vi "Autonomous Independent.vi"() -> ()   [LabVIEW 2019]
doc: "This VI is called when autonomous begins, and will automatically be terminated when autonomous ends. You can carry out timed or sensor driven robot movement independently without needing to return to the caller."
uses:
  <vilib>/Rock Robotics/WPI/Utilities/WPI_GetSetVariantRefNum.vi
  <vilib>/Rock Robotics/Network Tables/NT Write Numeric Array.vi
  <vilib>/Rock Robotics/WPI/RobotDrive/WPI_RobotDriveArcadeDrive_Standard(NoSaturation).vi
  <vilib>/Rock Robotics/Network Tables/NT Read String.vi
  <vilib>/Rock Robotics/WPI/Ultrasonic/WPI_SonarSRF04DigitalRefNum Registry Get.vi
  <vilib>/Rock Robotics/WPI/Ultrasonic/WPI_SonarSRF04DigitalGetRange.vi
  <vilib>/Rock Robotics/WPI/Ultrasonic/WPI_UltrasonicRangeUnits.ctl
panel:
  out "Ultrasonic 2":dbl
  out "Ultrasonic":dbl
  out "Degrees 2":dbl(knob) scale=0.0..360.0
  out "Degrees":dbl(knob) scale=0.0..360.0
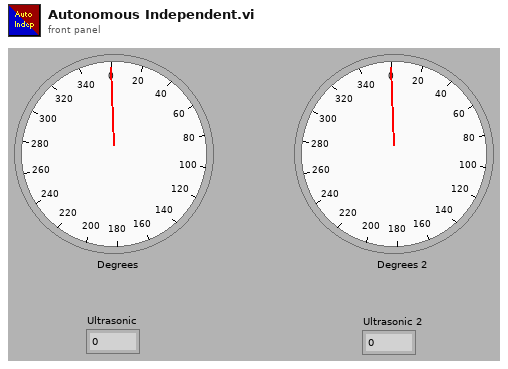
[diagram p1: front panel]
types:
  T1 = typedef "WPI_JoystickDevRef.ctl" = cluster{"Device":T2}
  T2 = typedef "WPI_JoystickDeviceEnum.ctl" = enum16{"USB 0", "USB 1", "USB 2", "USB 3", "USB 4", "USB 5"}
  T3 = typedef "WPI_UltrasonicRangeUnits.ctl" = enum16{"inches", "mm"}
  T4 = typedef "WPI_RobotDriveDevRef.ctl" = cluster{"DevStatus":errorcluster, "Motors[]":T5[], "Square Inputs":bool, "Max Output":dbl}
  T5 = typedef "WPI_MotorControlDeviceRef.ctl" = cluster{"DeviceStatus":errorcluster, "Type":T6, "PWM":cluster{"PWM Channel":T7, "DeadBand":T8}, "CAN":cluster{"Device Number":u8, "SetOutput VI Ref":variant, "GetOutput VI Ref":variant, "Enable VI Ref":variant, "Disable VI Ref":variant, "Data":variant}, "Invert":bool, "DIO PWM":cluster{"PWM \"Enable\" Channel":T7, "DIOChannel":T9, "PWM Rate":dbl}}
  T6 = typedef "WPI_MotorControlType.ctl" = enum16{"PWM", "CAN", "DIO PWM"}
  T7 = typedef "FPGA_DIOPWMChannel.ctl" = enum8{"PWM 0", "PWM 1", "PWM 2", "PWM 3", "PWM 4", "PWM 5", "PWM 6", "PWM 7", "PWM 8", "PWM 9", "PWM MXP 0", "PWM MXP 1", "PWM MXP 2", "PWM MXP 3", "PWM MXP 4", "PWM MXP 5", "PWM MXP 6", "PWM MXP 7", "PWM MXP 8", "PWM MXP 9", "Invalid"}
  T8 = typedef "WPI_PWMDeadband.ctl" = cluster{"Name":string, "maxPositivePwm":i32, "minPositivePwm":i32, "centerPwm":i32, "maxNegativePwm":i32, "minNegativePwm":i32, "angularRange":u16}
  T9 = typedef "FPGA_DIOChannel.ctl" = enum8{"DIO 0", "DIO 1", "DIO 2", "DIO 3", "DIO 4", "DIO 5", "DIO 6", "DIO 7", "DIO 8", "DIO 9", "DIO MXP 0", "DIO MXP 1", "DIO MXP 2", "DIO MXP 3", "DIO MXP 4", "DIO MXP 5", "DIO MXP 6", "DIO MXP 7", "DIO MXP 8", "DIO MXP 9", "DIO MXP 10", "DIO MXP 11", "DIO MXP 12", "DIO MXP 13", "DIO MXP 14", "DIO MXP 15", "SPI Port CS1", "SPI Port CS2", "SPI Port CS3", "SPI Port MISO", "SPI Port MOSI", "Invalid"}
  T10 = typedef "WPI_I2CDevRef.ctl" = cluster{"DevStatus":errorcluster, "Device Address":u8, "Handle":i32, "I2C Bus":T11}
  T11 = typedef "i2c_bus.ctl" = enum16{"I2C On-Board", "I2C MXP", "Invalid"}
  T12 = typedef "WPI_UltrasonicDeviceRef.ctl" = cluster{"DevStatus":errorcluster, "Ping Channel":T9, "Echo Channel":T9, "CntIndex":T13}
  T13 = typedef "FPGA_CounterCtrSystemIndex.ctl" = enum8{"Ctr 0", "Ctr 1", "Ctr 2", "Ctr 3", "Ctr 4", "Ctr 5", "Ctr 6", "Ctr 7", "Invalid"}
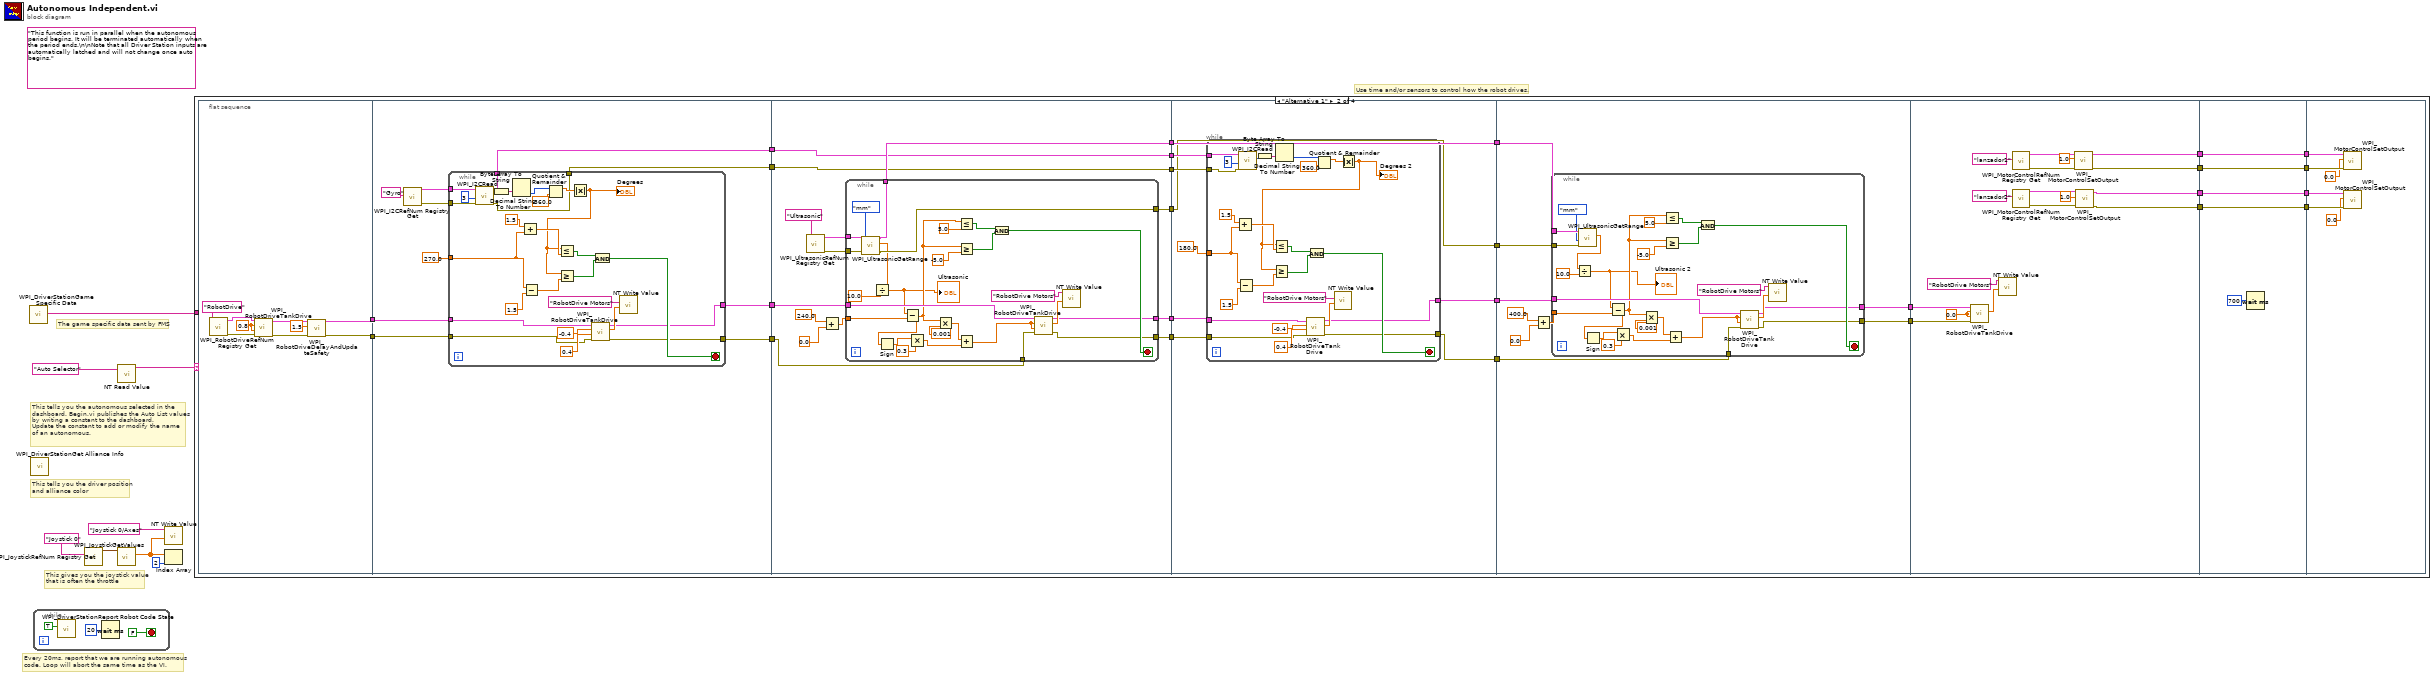
[diagram p0: block diagram]
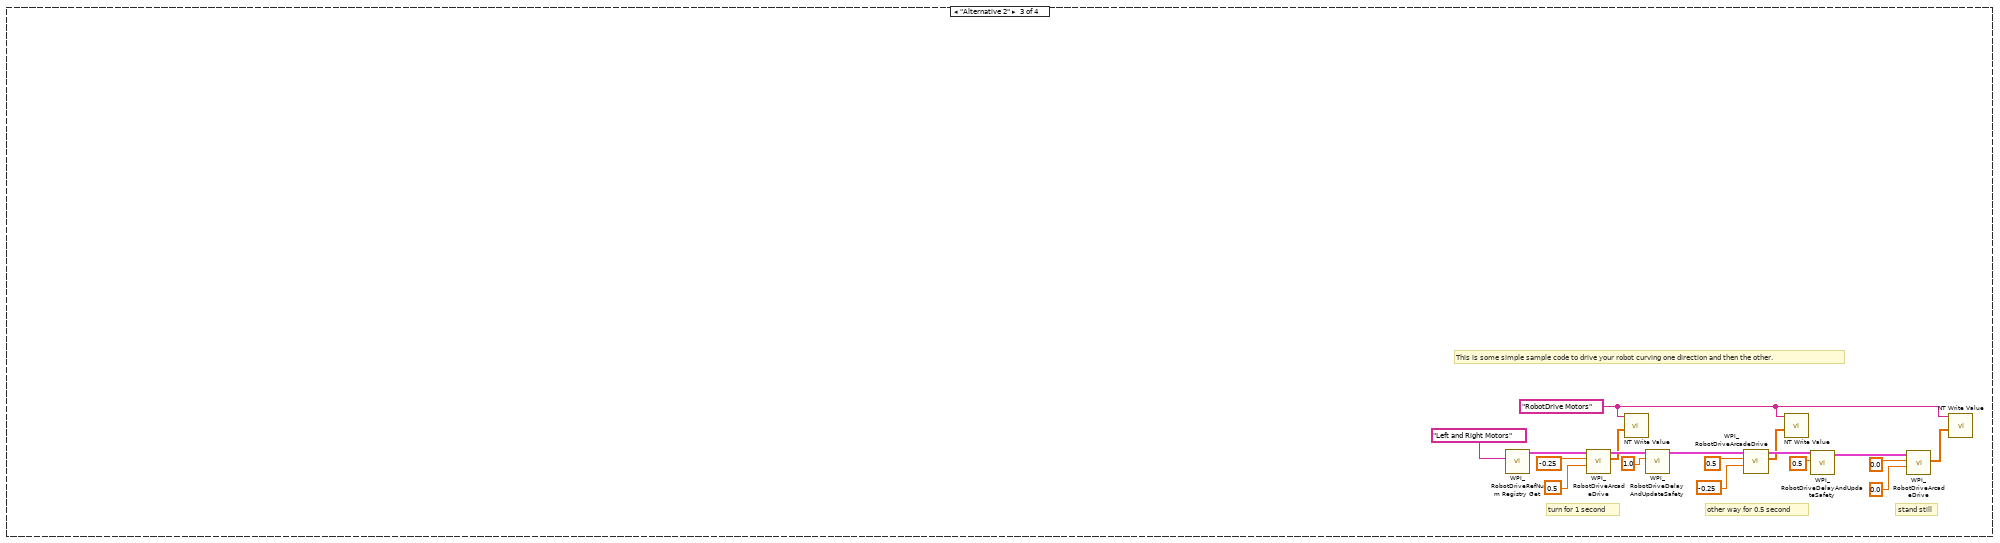
[diagram p3: hidden frame]
diagram:
  (unwired) "This function is run in parallel when the autonomous period begins. It will be terminated automatically when the period ends.\n\nNote that all Driver Station inputs are automatically latched and will not change once auto begins."
  # "The game specific data sent by FMS"
  # "This tells you the autonomous selected in the \ndashboard. Begin.vi publishes the Auto List values\nby writing a constant to the dashboard.\nUpdate the constant to add or modify the name\nof an autonomous."
  # "Every 20ms, report that we are running autonomous\ncode. Loop will abort the same time as the VI."
  # "This gives you the joystick value\nthat is often the throttle"
  # "Use time and/or sensors to control how the robot drives."
  # "This tells you the driver position\nand alliance color"
  n1 = call <vilib>:"WPI_DriverStationGame Specific Data.vi"() -> ("Game Specific Data"=w1:string)  [unwired: 11 in]
  n2 = call <vilib>:"WPI_DriverStationGet Alliance Info.vi"() -> ()  [unwired: 12 out]
  n3 = while {
    stop <- FALSE stop-if-true
    n4 = call <vilib>:"WPI_DriverStationReport Robot Code State.vi"("Autonomous"=TRUE) -> ()  [unwired: 10 in, 1 out]
    n5 = Wait (ms)(milliseconds to wait=u32 20) -> ()  [unwired: 1 out]
  }
  n6 = call <vilib>:"WPI_JoystickRefNum Registry Get.vi"("refnum name"="Joystick 0") -> ("JoystickDevRef"=w7:T1)  [unwired: 1 in, 9 out]
  n7 = call <vilib>:"WPI_JoystickGetValues.vi"("JoystickDevRef"=w7) -> ("Axes"=w3:dbl[])  [unwired: 6 in, 4 out]
  n8 = call-poly <vilib>:"NT Read Value.vi"("Name"="Auto Selector") -> ("String"=w4:string)  [unwired: 9 in, 1 out]
  n9 = call-poly <vilib>:"NT Write Value.vi"("Numeric Array"=w3, "Name"="Joystick 0/Axes") -> ()  [unwired: 9 in, 1 out]
  n10 = Index Array(array=w3, index=2) -> ()  [unwired: 1 out]
  n11 = case shown="\"Alternative 1\"" w4 {
    tunnel: w1 -> [_ _ _ _]
    frame Default {
      # "You can put your main auto here, or you can right-click on the case and make any\nother frame be the default case."
      # "This is the frame that will execute if no selection is made, or if it is not recognized"
    }
    frame "Alternative 1" {
      n12 = flat-sequence {
        tunnel: [w38] -> w15
        tunnel: [w39] -> w14
        tunnel: [w55] -> w37
        tunnel: [w54] -> w36
        tunnel: w15 -> [w50]
        tunnel: w14 -> [w49]
        tunnel: [w48] -> w13
        tunnel: [w47] -> w12
        tunnel: w37 -> [w91]
        tunnel: w36 -> [w90]
        tunnel: [w89] -> w35
        tunnel: [w88] -> w34
        tunnel: [w85] -> w33
        tunnel: [w84] -> w32
        tunnel: [w87] -> w31
        tunnel: [w86] -> w30
        tunnel: w13 -> [w85]
        tunnel: w12 -> [w84]
        tunnel: w35 -> [w133]
        tunnel: w34 -> [w132]
        tunnel: w33 -> [w130]
        tunnel: w32 -> [w129]
        tunnel: [w128] -> w29
        tunnel: [w127] -> w28
        tunnel: [w126] -> w27
        tunnel: w31 -> [w126]
        tunnel: [w125] -> w26
        tunnel: w30 -> [w125]
        tunnel: w29 -> [w167]
        tunnel: w28 -> [w163]
        tunnel: w27 -> [w162]
        tunnel: w26 -> [w161]
        tunnel: [w160] -> w25
        tunnel: [w159] -> w24
        tunnel: w25 -> [w199]
        tunnel: w24 -> [w198]
        tunnel: [w196] -> w23
        tunnel: [w195] -> w22
        tunnel: [w194] -> w21
        tunnel: [w193] -> w20
        tunnel: [w213] -> w19
        tunnel: w23 -> [w213]
        tunnel: [w212] -> w18
        tunnel: w22 -> [w212]
        tunnel: [w211] -> w17
        tunnel: w21 -> [w211]
        tunnel: [w210] -> w16
        tunnel: w20 -> [w210]
        tunnel: w19 -> [w220]
        tunnel: w18 -> [w219]
        tunnel: w17 -> [w218]
        tunnel: w16 -> [w217]
        frame #0 {
          w43 = 0.8 ("Left axis value")
          n13 = call <vilib>:"WPI_RobotDriveRefNum Registry Get.vi"("refnum name"="RobotDrive") -> ("error out"=w41:errorcluster, "RobotDriveDevRef"=w42:T4)  [unwired: 9 in]
          n14 = call <vilib>:"WPI_RobotDriveTankDrive.vi"("error in (no error)"=w41, "Right axis value"=w43, "Left axis value"=w43, "RobotDriveDevRef"=w42) -> ("error out"=w44:errorcluster, "RobotDriveDevRef"=w45:T4)  [unwired: 5 in, 1 out]
          n15 = call <vilib>:"WPI_RobotDriveDelayAndUpdateSafety.vi"("error in (no error)"=w44, "Delay (s)"=1.5, "RobotDriveDevRef"=w45) -> ("error out"=w38:errorcluster, "RobotDriveDevRef 2"=w39:T4)  [unwired: 7 in]
        }
        frame #1 {
          n16 = call <vilib>:"WPI_I2CRefNum Registry Get.vi"("refnum name"="Gyro") -> ("error out"=w52:errorcluster, "I2CDevRef"=w51:T10)  [unwired: 9 in]
          n17 = while {
            tunnel: 270.0 ("y") -> [w76]
            tunnel: [w69] -> w55
            tunnel: [w68] -> w54
            tunnel: w52 -> [w65]
            tunnel: w51 -> [w64]
            tunnel: w50 -> [w60]
            tunnel: w49 -> [w59]
            tunnel: [w58] -> w48
            tunnel: [w57] -> w47
            stop <- w79 stop-if-true
            n18 = call <vilib>:"WPI_I2CRead.vi"("error in (no error)"=w65, "I2CBytesToRead"=u8 3, "I2CDevRef"=w64) -> ("error out"=w57:errorcluster, "Data Out"=w62:u8[], "I2CDevRef"=w58:T10)  [unwired: 6 in]
            n19 = Byte Array To String(unsigned byte array=w62) -> (string=w66:string)
            n20 = Decimal String To Number(string=w66) -> (number=w61:i32)  [unwired: 2 in, 1 out]
            n21 = Add(x=1.5 ("y"), y=w76) -> (x+y=w72:dbl)
            n22 = Subtract(x=w76, y=1.5 ("x")) -> (x-y=w73:dbl)
            n23 = Quotient & Remainder(x=w61, y=360.0) -> (x-y*floor(x/y)=w70:dbl)  [unwired: 1 out]
            n24 = Absolute Value(x=w70) -> (abs(x)=w67:dbl)
            "Degrees" <- w67
            n25 = Less Or Equal?(x=w67, y=w72) -> (x <= y?=w74:bool)
            n26 = Greater Or Equal?(x=w67, y=w73) -> (x >= y?=w75:bool)
            n27 = call <vilib>:"WPI_RobotDriveTankDrive.vi"("error in (no error)"=w60, "Right axis value"=0.4 ("X axis value"), "Left axis value"=-0.4 ("X axis value"), "RobotDriveDevRef"=w59) -> ("error out"=w68:errorcluster, "Motor Values"=w83:dbl[], "RobotDriveDevRef"=w69:T4)  [unwired: 5 in]
            n28 = And(x=w74, y=w75) -> (x .and. y?=w79:bool)
            n29 = call-poly <vilib>:"NT Write Value.vi"("Numeric Array"=w83, "Name"="RobotDrive Motors") -> ()  [unwired: 9 in, 1 out]
          }
        }
        frame #2 {
          n30 = call-poly <vilib>:"WPI_UltrasonicRefNum Registry Get.vi"("refnum name"="Ultrasonic") -> ("error out"=w96:errorcluster, "SonarSRF04DevRef"=w95:T12)  [unwired: 9 in]
          n31 = Add(x=240.0 ("y"), y=0.0) -> (x+y=w92:dbl)
          n32 = while {
            tunnel: w96 -> [w105]
            tunnel: w95 -> [w104]
            tunnel: w92 -> [w124]
            tunnel: w91 -> [w119]
            tunnel: w90 -> [w115]
            tunnel: [w107] -> w89
            tunnel: [w106] -> w88
            tunnel: [w102] -> w87
            tunnel: [w101] -> w86
            stop <- w111 stop-if-true
            n33 = call-poly <vilib>:"WPI_UltrasonicGetRange.vi"("error in (no error)"=w105, "Range Units"=WPI_UltrasonicRangeUnits."mm", "SonarSRF04DevRef"=w104) -> ("error out"=w101:errorcluster, "Distance"=w100:dbl, "SonarSRF04DevRef"=w102:T12)  [unwired: 6 in]
            n34 = Divide(x=w100, y=10.0) -> (x/y=w98:dbl)
            "Ultrasonic" <- w98
            n35 = Subtract(x=w98, y=w124) -> (x-y=w108:dbl)
            n36 = Sign(1:w108) -> (0:w118:dbl)
            n37 = Multiply(x=w118, y=0.3) -> (x*y=w116:dbl)
            n38 = Multiply(x=w108, y=0.001) -> (x*y=w122:dbl)
            n39 = Less Or Equal?(x=w108, y=5.0 ("x")) -> (x <= y?=w113:bool)
            n40 = Greater Or Equal?(x=w108, y=-5.0 ("x")) -> (x >= y?=w112:bool)
            n41 = Add(x=w122, y=w116) -> (x+y=w114:dbl)
            n42 = And(x=w113, y=w112) -> (x .and. y?=w111:bool)
            n43 = call <vilib>:"WPI_RobotDriveTankDrive.vi"("error in (no error)"=w115, "Right axis value"=w114, "Left axis value"=w114, "RobotDriveDevRef"=w119) -> ("error out"=w107:errorcluster, "Motor Values"=w121:dbl[], "RobotDriveDevRef"=w106:T4)  [unwired: 5 in]
            n44 = call-poly <vilib>:"NT Write Value.vi"("Numeric Array"=w121, "Name"="RobotDrive Motors") -> ()  [unwired: 9 in, 1 out]
          }
        }
        frame #3 {
          n45 = while {
            tunnel: w132 -> [w154]
            tunnel: w133 -> [w153]
            tunnel: 180.0 ("y") -> [w149]
            tunnel: [w142] -> w128
            tunnel: [w141] -> w127
            tunnel: w130 -> [w137]
            tunnel: w129 -> [w136]
            stop <- w152 stop-if-true
            n46 = Add(x=1.5 ("y"), y=w149) -> (x+y=w145:dbl)
            n47 = Subtract(x=w149, y=1.5 ("x")) -> (x-y=w146:dbl)
            n48 = call <vilib>:"WPI_I2CRead.vi"("error in (no error)"=w136, "I2CBytesToRead"=u8 3, "I2CDevRef"=w137) -> ("Data Out"=w138:u8[])  [unwired: 6 in, 2 out]
            n49 = Byte Array To String(unsigned byte array=w138) -> (string=w140:string)
            n50 = Decimal String To Number(string=w140) -> (number=w135:i32)  [unwired: 2 in, 1 out]
            n51 = call <vilib>:"WPI_RobotDriveTankDrive.vi"("error in (no error)"=w153, "Right axis value"=0.4 ("X axis value"), "Left axis value"=-0.4 ("X axis value"), "RobotDriveDevRef"=w154) -> ("error out"=w141:errorcluster, "Motor Values"=w158:dbl[], "RobotDriveDevRef"=w142:T4)  [unwired: 5 in]
            n52 = Quotient & Remainder(x=w135, y=360.0) -> (x-y*floor(x/y)=w143:dbl)  [unwired: 1 out]
            n53 = call-poly <vilib>:"NT Write Value.vi"("Numeric Array"=w158, "Name"="RobotDrive Motors") -> ()  [unwired: 9 in, 1 out]
            n54 = Absolute Value(x=w143) -> (abs(x)=w134:dbl)
            "Degrees 2" <- w134
            n55 = Less Or Equal?(x=w134, y=w145) -> (x <= y?=w147:bool)
            n56 = Greater Or Equal?(x=w134, y=w146) -> (x >= y?=w148:bool)
            n57 = And(x=w147, y=w148) -> (x .and. y?=w152:bool)
          }
        }
        frame #4 {
          n58 = Add(x=400.0 ("y"), y=0.0) -> (x+y=w164:dbl)
          n59 = while {
            tunnel: w161 -> [w173]
            tunnel: w162 -> [w172]
            tunnel: w164 -> [w192]
            tunnel: w167 -> [w187]
            tunnel: w163 -> [w183]
            tunnel: [w175] -> w160
            tunnel: [w174] -> w159
            stop <- w179 stop-if-true
            n60 = call-poly <vilib>:"WPI_UltrasonicGetRange.vi"("error in (no error)"=w173, "Range Units"=WPI_UltrasonicRangeUnits."mm", "SonarSRF04DevRef"=w172) -> ("Distance"=w170:dbl)  [unwired: 6 in, 2 out]
            n61 = Divide(x=w170, y=10.0) -> (x/y=w168:dbl)
            "Ultrasonic 2" <- w168
            n62 = Subtract(x=w168, y=w192) -> (x-y=w176:dbl)
            n63 = Sign(1:w176) -> (0:w186:dbl)
            n64 = Multiply(x=w186, y=0.3) -> (x*y=w184:dbl)
            n65 = Multiply(x=w176, y=0.001) -> (x*y=w190:dbl)
            n66 = Less Or Equal?(x=w176, y=5.0 ("x")) -> (x <= y?=w181:bool)
            n67 = Greater Or Equal?(x=w176, y=-5.0 ("x")) -> (x >= y?=w180:bool)
            n68 = Add(x=w190, y=w184) -> (x+y=w182:dbl)
            n69 = And(x=w181, y=w180) -> (x .and. y?=w179:bool)
            n70 = call <vilib>:"WPI_RobotDriveTankDrive.vi"("error in (no error)"=w183, "Right axis value"=w182, "Left axis value"=w182, "RobotDriveDevRef"=w187) -> ("error out"=w174:errorcluster, "Motor Values"=w189:dbl[], "RobotDriveDevRef"=w175:T4)  [unwired: 5 in]
            n71 = call-poly <vilib>:"NT Write Value.vi"("Numeric Array"=w189, "Name"="RobotDrive Motors") -> ()  [unwired: 9 in, 1 out]
          }
        }
        frame #5 {
          w197 = 0.0 ("Left axis value")
          n72 = call <vilib>:"WPI_RobotDriveTankDrive.vi"("error in (no error)"=w198, "Right axis value"=w197, "Left axis value"=w197, "RobotDriveDevRef"=w199) -> ("Motor Values"=w201:dbl[])  [unwired: 5 in, 2 out]
          n73 = call-poly <vilib>:"NT Write Value.vi"("Numeric Array"=w201, "Name"="RobotDrive Motors") -> ()  [unwired: 9 in, 1 out]
          n74 = call <vilib>:"WPI_MotorControlRefNum Registry Get.vi"("refnum name"="lanzador1") -> ("error out"=w208:errorcluster, "MotorControlDevRef"=w209:T5)  [unwired: 9 in]
          n75 = call <vilib>:"WPI_MotorControlRefNum Registry Get.vi"("refnum name"="lanzador2") -> ("error out"=w204:errorcluster, "MotorControlDevRef"=w205:T5)  [unwired: 9 in]
          n76 = call <vilib>:"WPI_MotorControlSetOutput.vi"("error in (no error)"=w208, "Output"=1.0, "MotorControlDevRef"=w209) -> ("error out"=w193:errorcluster, "MotorControlDevRef"=w196:T5)  [unwired: 6 in, 1 out]
          n77 = call <vilib>:"WPI_MotorControlSetOutput.vi"("error in (no error)"=w204, "Output"=1.0, "MotorControlDevRef"=w205) -> ("error out"=w194:errorcluster, "MotorControlDevRef"=w195:T5)  [unwired: 6 in, 1 out]
        }
        frame #6 {
          n78 = Wait (ms)(milliseconds to wait=u32 700) -> ()  [unwired: 1 out]
        }
        frame #7 {
          n79 = call <vilib>:"WPI_MotorControlSetOutput.vi"("error in (no error)"=w217, "Output"=0.0, "MotorControlDevRef"=w220) -> ()  [unwired: 6 in, 3 out]
          n80 = call <vilib>:"WPI_MotorControlSetOutput.vi"("error in (no error)"=w218, "Output"=0.0, "MotorControlDevRef"=w219) -> ()  [unwired: 6 in, 3 out]
        }
      }
    }
    frame "Alternative 2" {
      w222 = "RobotDrive Motors" ("Name")
      # "This is some simple sample code to drive your robot curving one direction and then the other."
      # "stand still"
      # "other way for 0.5 second"
      # "turn for 1 second"
      n81 = call <vilib>:"WPI_RobotDriveRefNum Registry Get.vi"("refnum name"="Left and Right Motors") -> ("RobotDriveDevRef"=w238:T4)  [unwired: 1 in, 9 out]
      n82 = call-poly <vilib>:"WPI_RobotDriveArcadeDrive.vi"("Y axis value"=0.5 ("X axis value"), "X axis value"=-0.25, "RobotDriveDevRef"=w238) -> ("Motor Values"=w221:dbl[], "RobotDriveDevRef"=w231:T4)  [unwired: 1 in, 6 out]
      n83 = call-poly <vilib>:"NT Write Value.vi"("Numeric Array"=w221, "Name"=w222) -> ()  [unwired: 9 in, 1 out]
      n84 = call <vilib>:"WPI_RobotDriveDelayAndUpdateSafety.vi"("Delay (s)"=1.0, "RobotDriveDevRef"=w231) -> ("RobotDriveDevRef 2"=w232:T4)  [unwired: 8 in, 1 out]
      n85 = call-poly <vilib>:"WPI_RobotDriveArcadeDrive.vi"("Y axis value"=-0.25 ("X axis value"), "X axis value"=0.5, "RobotDriveDevRef"=w232) -> ("Motor Values"=w223:dbl[], "RobotDriveDevRef"=w233:T4)  [unwired: 1 in, 6 out]
      n86 = call-poly <vilib>:"NT Write Value.vi"("Numeric Array"=w223, "Name"=w222) -> ()  [unwired: 9 in, 1 out]
      n87 = call <vilib>:"WPI_RobotDriveDelayAndUpdateSafety.vi"("Delay (s)"=0.5, "RobotDriveDevRef"=w233) -> ("RobotDriveDevRef 2"=w234:T4)  [unwired: 8 in, 1 out]
      n88 = call-poly <vilib>:"WPI_RobotDriveArcadeDrive.vi"("Y axis value"=0.0 ("X axis value"), "X axis value"=0.0, "RobotDriveDevRef"=w234) -> ("Motor Values"=w224:dbl[])  [unwired: 1 in, 7 out]
      n89 = call-poly <vilib>:"NT Write Value.vi"("Numeric Array"=w224, "Name"=w222) -> ()  [unwired: 9 in, 1 out]
    }
    frame "Your Turn" {
    }
  }
